vi "CalVEIN Main.vi"() -> ()   [LabVIEW 2017]
uses:
  Type Defs/Sensor Data.ctl
  Type Defs/Boxcar.ctl
panel:
  out "45% 2":string="31.00 °C"
  out "45%":string="31.10 °C"
  in  "Box cooler":bool
  out "NewVal":bool
  out "Ready To Fire Flag":bool
  out "Firing State":string[](array[string])=["System Is Not Armed", "", "", "", "", " "]
  in  "Arm Flag":bool
  in  "Sample Rate (secs)":u32=1000
  out "Burn Time\nCountdown (secs)":string="0.00"
  out "Boxcar Data":T1={"AI Sensor Data"={"Sensor Array"=[{"Description"="P2 - LOX Tank Pressure", "Last Reading"="-1.72", "Coefs"=[0.0, 5000.0], "Eng Units"="psig"}, {"Description"="P3 - Fuel Tank Pressure", "Last Reading"="-1.03", "Coefs"=[0.0, 5000.0], "Eng Units"="psig"}, {"Description"="P1 - Chamber Pressure", "Last Reading"="-1.17", "Coefs"=[0.0, 5000.0], "Eng Units"="psig"}, {"Description"="Not Used", "Last Reading"="0.00", "Coefs"=[0.0, 0.0], "Eng Units"="psig"}, {"Description"="P5- DOME Reg.", "Last Reading"="-1.58", "Coefs"=[0.0, 5000.0], "Eng Units"="psig"}, {"Description"="Not Use", "Last Reading"="0.00", "Coefs"=[0.0, 0.0], "Eng Units"="psig"}, {"Description"="P4- High Pressure Tank", "Last Reading"="-1.56", "Coefs"=[0.0, 10000.0], "Eng Units"="psig"}, {"Description"="P7 - Gnd High Pressure", "Last Reading"="-4.62", "Coefs"=[0.0, 10000.0], "Eng Units"="psig"}, {"Description"="P6 - GHE Fill Pressure", "Last Reading"="2.98", "Coefs"=[0.0, 5000.0], "Eng Units"="psig"}, {"Description"="P8 - Pneumatics Pressure", "Last Reading"="0.32", "Coefs"=[0.0, 5000.0], "Eng Units"="psig"}, {"Description"="Not Used", "Last Reading"="0.00", "Coefs"=[0.0, 0.0], "Eng Units"=""}, {"Description"="Not Used", "Last Reading"="0.00", "Coefs"=[0.0, 0.0], "Eng Units"=""}, {"Description"="Not Used", "Last Reading"="0.00", "Coefs"=[0.0, 0.0], "Eng Units"=""}, {"Description"="Not Used", "Last Reading"="0.00", "Coefs"=[0.0, 0.0], "Eng Units"=""}, {"Description"="Not Used", "Last Reading"="0.00", "Coefs"=[0.0, 0.0], "Eng Units"=""}, {"Description"="Not Used", "Last Reading"="0.00", "Coefs"=[0.0, 0.0], "Eng Units"=""}, {"Description"="QD Sep Indication", "Last Reading"="5.09", "Coefs"=[0.0, 1.0], "Eng Units"="On/Off"}, {"Description"="Lift Off Indicator", "Last Reading"="5.09", "Coefs"=[0.0, 1.0], "Eng Units"="On/Off"}, {"Description"="Main Valve Open Indicator", "Last Reading"="1.79", "Coefs"=[0.0, 1.0], "Eng Units"="On/Off"}, {"Description"="Main Valve Closed Indicator", "Last Reading"="1.76", "Coefs"=[0.0, 1.0], "Eng Units"="On/Off"}, {"Description"="Load Cell 1 - Veh Gross Weight", "Last Reading"="0.13", "Coefs"=[-122.0, 8333.3], "Eng Units"="lbf"}, {"Description"="Load Cell 2 - - Veh Gross Weight", "Last Reading"="-2.48", "Coefs"=[0.0, 8333.33], "Eng Units"="lbf"}, {"Description"="Not Used", "Last Reading"="0.00", "Coefs"=[0.0, 0.0], "Eng Units"=""}, {"Description"="Not Used", "Last Reading"="0.00", "Coefs"=[0.0, 0.0], "Eng Units"=""}, {"Description"="", "Last Reading"="0.00", "Coefs"=[], "Eng Units"=""}, {"Description"="", "Last Reading"="0.00", "Coefs"=[], "Eng Units"=""}, {"Description"="", "Last Reading"="0.00", "Coefs"=[], "Eng Units"=""}, {"Description"="", "Last Reading"="0.00", "Coefs"=[], "Eng Units"=""}, {"Description"="", "Last Reading"="0.00", "Coefs"=[], "Eng Units"=""}, {"Description"="", "Last Reading"="0.00", "Coefs"=[], "Eng Units"=""}, {"Description"="", "Last Reading"="0.00", "Coefs"=[], "Eng Units"=""}, {"Description"="", "Last Reading"="0.00", "Coefs"=[], "Eng Units"=""}]}, "TC Array"=[31.195067822, 31.09588569350001, 31.09588569350001, 30.99670356499999, 31.195067822, 31.09588569350001, 31.09588569350001, 1369.6815, 1369.6815, 1369.6815, 1369.6815, 1369.6815, 1369.6815, 1369.6815]}
  out "?":string="3.07 psig"
  out "Log Refnum":refnum<file>
  out "Log Epoch":u32
  out "Log Number":i32=123
  in  "Data Log Flag":bool
  out "File Path":path
  out "Eng Data & Units":string[](array[string])=["-1.67 psig", "-1.03 psig", "-1.17 psig", "0.00 psig", "-1.58 psig", "0.00 psig", "-1.56 psig", "-4.62 psig", "3.07 psig", "0.32 psig", "0.00 ", "0.00 ", "0.00 ", "0.00 ", "0.00 ", "0.00 ", "5.09 On/Off", "5.09 On/Off", "1.79 On/Off", "1.75 On/Off", "0.13 lbf", "-2.48 lbf", "0.00 ", "0.00 ", "0.00 ", "0.00 ", "0.00 ", "0.00 ", "0.00 ", "0.00 ", "0.00 ", "0.00 "]
  out "TC String Array":string[](array[string])=["31.20 °C", "31.10 °C", "31.10 °C", "31.00 °C", "31.20 °C", "31.10 °C", "31.10 °C", "1369.68 °C", "1369.68 °C", "1369.68 °C", "1369.68 °C", "1369.68 °C", "1369.68 °C", "1369.68 °C"]
  in  "Data Log Button":bool
  in  "Sequence Abort":bool
  out "Igniter Abort":bool
  out "Elapsed Time":u32=10554
  in  "Auto Sequence":bool
  in  "Auto Sequence Flag":bool
  out "Epoch":u32=5746771
  out "Countdown (secs)":i32
  in  "MV Open Start":dbl
  in  "Burn Time":dbl=3.0
  in  "Igniter Start":dbl=-3.0
  in  "Countdown":dbl=-10.0
  in  "Igniter Minimum\nTemp (°C)":dbl=200.0
  in  "Auto Switch":bool
  out "?":string="1369.68 °C"
  out "Thermometer 2":dbl(slide)=1369.6815 scale=0.0..1000.0
  out "Thermometer":dbl(slide)=1369.6815 scale=0.0..1000.0
  out "Igniter Temp (°C)":string="1369.68 °C"
  out "?":string="31.20 °C"
  out "30%":string="31.10 °C"
  out "QD Sep Indicator":bool=TRUE
  out "Liftoff Indicator":bool=TRUE
  out "MV Closed Ind":bool
  out "MV Open Ind":bool
  out "?":string="0.13 lbf"
  out "?":string="0.32 psig"
  out "?":string="-4.62 psig"
  out "?":string="-1.58 psig"
  out "?":string="-1.56 psig"
  out "?":string="-1.17 psig"
  out "P3":string="-1.03 psig"
  in  "High Press":bool
  in  "High Press Vent":bool
  in  "MV Open":bool
  in  "MV Closed":bool
  out "P2":string="-1.67 psig"
  in  "Remote QD Sep":bool
  in  "GHe Fill":bool
  in  "Igniter Pwr":bool
  in  "Dome Reg":bool
  in  "Dome Vent":bool
  in  "Fuel Vent":bool
  in  "LOX Vent":bool
  out "Relay States":bool[](array[boolean])
  in  "stop":bool
  in  "AI Sensor Data":T2={"Sensor Array"=[{"Description"="P2 - LOX Tank Pressure", "Last Reading"="-1.67", "Coefs"=[0.0, 5000.0], "Eng Units"="psig"}, {"Description"="P3 - Fuel Tank Pressure", "Last Reading"="-1.03", "Coefs"=[0.0, 5000.0], "Eng Units"="psig"}, {"Description"="P1 - Chamber Pressure", "Last Reading"="-1.17", "Coefs"=[0.0, 5000.0], "Eng Units"="psig"}, {"Description"="Not Used", "Last Reading"="0.00", "Coefs"=[0.0, 0.0], "Eng Units"="psig"}, {"Description"="P5- DOME Reg.", "Last Reading"="-1.58", "Coefs"=[0.0, 5000.0], "Eng Units"="psig"}, {"Description"="Not Use", "Last Reading"="0.00", "Coefs"=[0.0, 0.0], "Eng Units"="psig"}, {"Description"="P4- High Pressure Tank", "Last Reading"="-1.56", "Coefs"=[0.0, 10000.0], "Eng Units"="psig"}, {"Description"="P7 - Gnd High Pressure", "Last Reading"="-4.62", "Coefs"=[0.0, 10000.0], "Eng Units"="psig"}, {"Description"="P6 - GHE Fill Pressure", "Last Reading"="3.07", "Coefs"=[0.0, 5000.0], "Eng Units"="psig"}, {"Description"="P8 - Pneumatics Pressure", "Last Reading"="0.32", "Coefs"=[0.0, 5000.0], "Eng Units"="psig"}, {"Description"="Not Used", "Last Reading"="0.00", "Coefs"=[0.0, 0.0], "Eng Units"=""}, {"Description"="Not Used", "Last Reading"="0.00", "Coefs"=[0.0, 0.0], "Eng Units"=""}, {"Description"="Not Used", "Last Reading"="0.00", "Coefs"=[0.0, 0.0], "Eng Units"=""}, {"Description"="Not Used", "Last Reading"="0.00", "Coefs"=[0.0, 0.0], "Eng Units"=""}, {"Description"="Not Used", "Last Reading"="0.00", "Coefs"=[0.0, 0.0], "Eng Units"=""}, {"Description"="Not Used", "Last Reading"="0.00", "Coefs"=[0.0, 0.0], "Eng Units"=""}, {"Description"="QD Sep Indication", "Last Reading"="5.09", "Coefs"=[0.0, 1.0], "Eng Units"="On/Off"}, {"Description"="Lift Off Indicator", "Last Reading"="5.09", "Coefs"=[0.0, 1.0], "Eng Units"="On/Off"}, {"Description"="Main Valve Open Indicator", "Last Reading"="1.79", "Coefs"=[0.0, 1.0], "Eng Units"="On/Off"}, {"Description"="Main Valve Closed Indicator", "Last Reading"="1.75", "Coefs"=[0.0, 1.0], "Eng Units"="On/Off"}, {"Description"="Load Cell 1 - Veh Gross Weight", "Last Reading"="0.13", "Coefs"=[-122.0, 8333.3], "Eng Units"="lbf"}, {"Description"="Load Cell 2 - - Veh Gross Weight", "Last Reading"="-2.48", "Coefs"=[0.0, 8333.33], "Eng Units"="lbf"}, {"Description"="Not Used", "Last Reading"="0.00", "Coefs"=[0.0, 0.0], "Eng Units"=""}, {"Description"="Not Used", "Last Reading"="0.00", "Coefs"=[0.0, 0.0], "Eng Units"=""}, {"Description"="", "Last Reading"="0.00", "Coefs"=[], "Eng Units"=""}, {"Description"="", "Last Reading"="0.00", "Coefs"=[], "Eng Units"=""}, {"Description"="", "Last Reading"="0.00", "Coefs"=[], "Eng Units"=""}, {"Description"="", "Last Reading"="0.00", "Coefs"=[], "Eng Units"=""}, {"Description"="", "Last Reading"="0.00", "Coefs"=[], "Eng Units"=""}, {"Description"="", "Last Reading"="0.00", "Coefs"=[], "Eng Units"=""}, {"Description"="", "Last Reading"="0.00", "Coefs"=[], "Eng Units"=""}, {"Description"="", "Last Reading"="0.00", "Coefs"=[], "Eng Units"=""}]}
  # "CSULB Launch Team Control System"
  # "Questions regrads this system please direct them to Thanh Truc Le truclee126@gmail.com"
  # "Autosequence\n Parameters"
  # "30%"
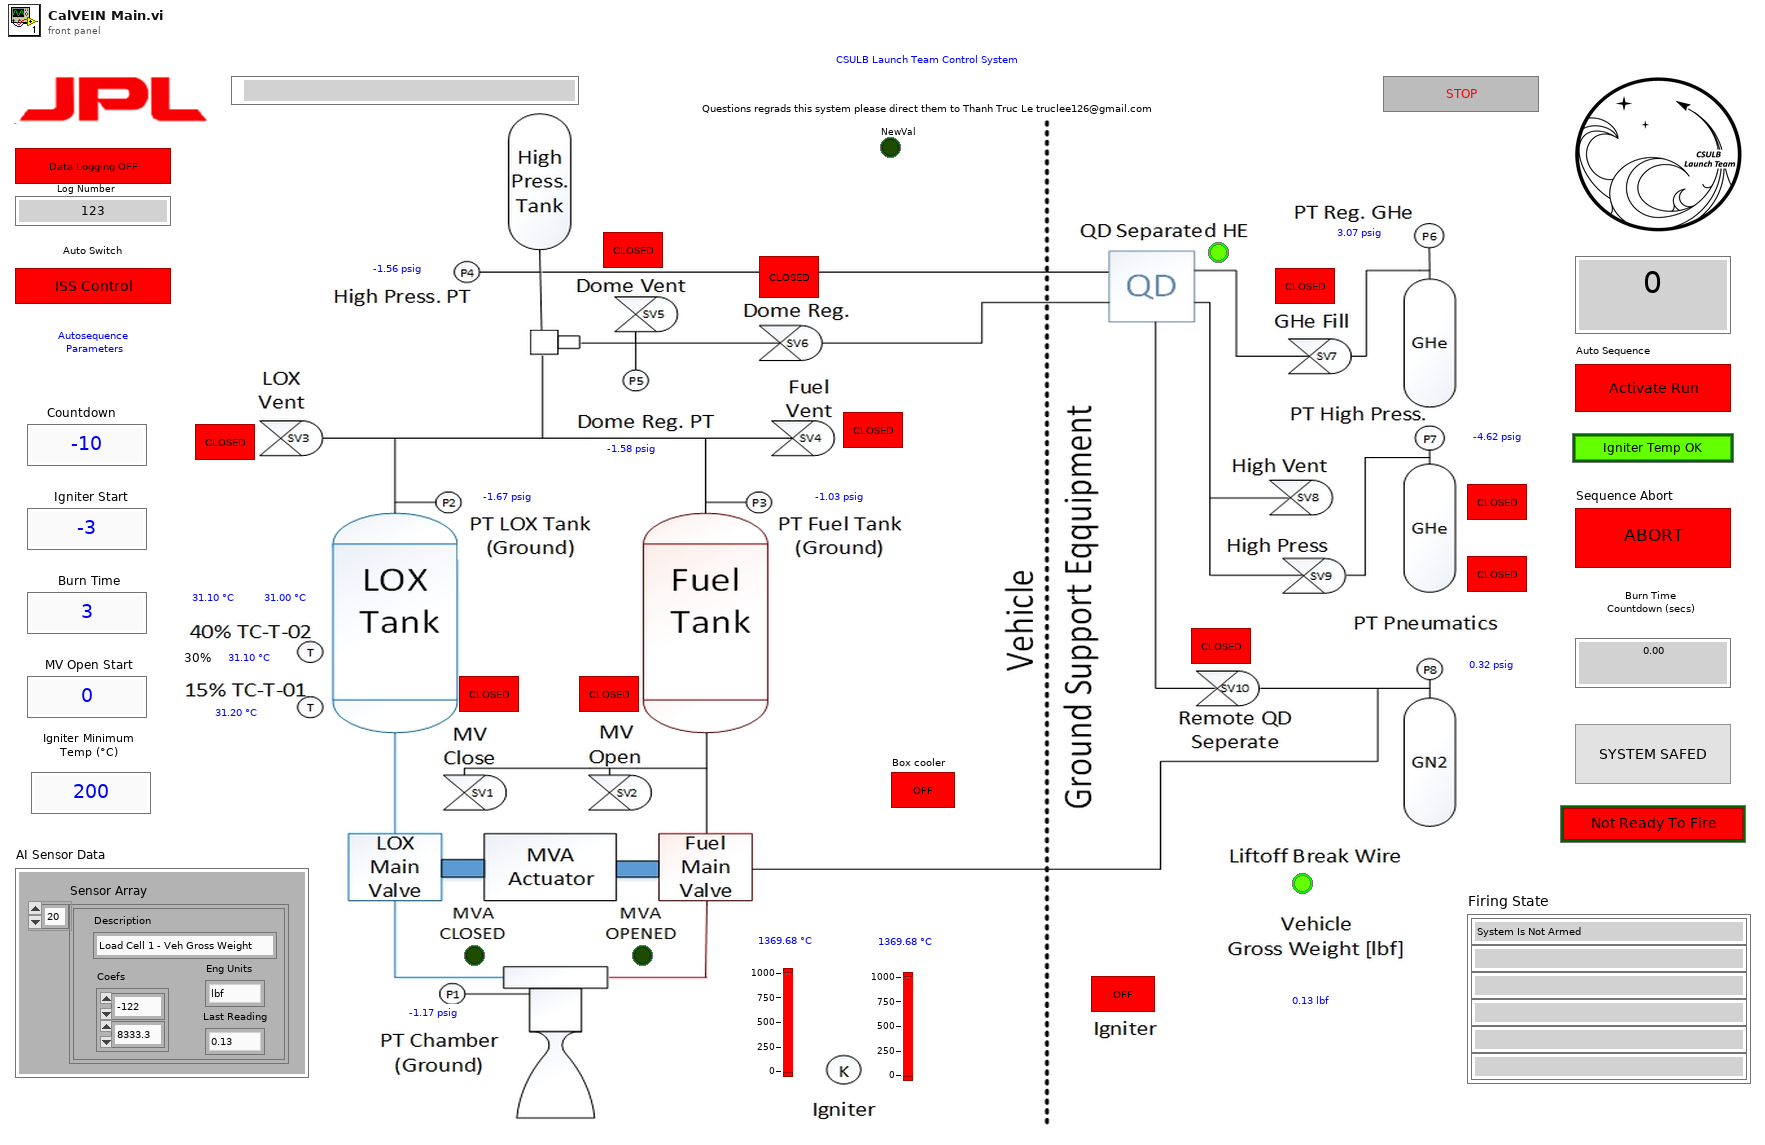
[diagram p1: front panel]
types:
  T1 = typedef "Boxcar.ctl" = cluster{"AI Sensor Data":T2, "TC Array":dbl[]}
  T2 = typedef "Sensor Data.ctl" = cluster{"Sensor Array":cluster{"Description":string, "Last Reading":string, "Coefs":dbl[], "Eng Units":string}[]}
  T3 = cluster{"Description":string, "Last Reading":string, "Coefs":dbl[], "Eng Units":string}[]
  T4 = enum16{"open", "replace", "create", "open or create", "replace or create", "replace or create with confirmation"}
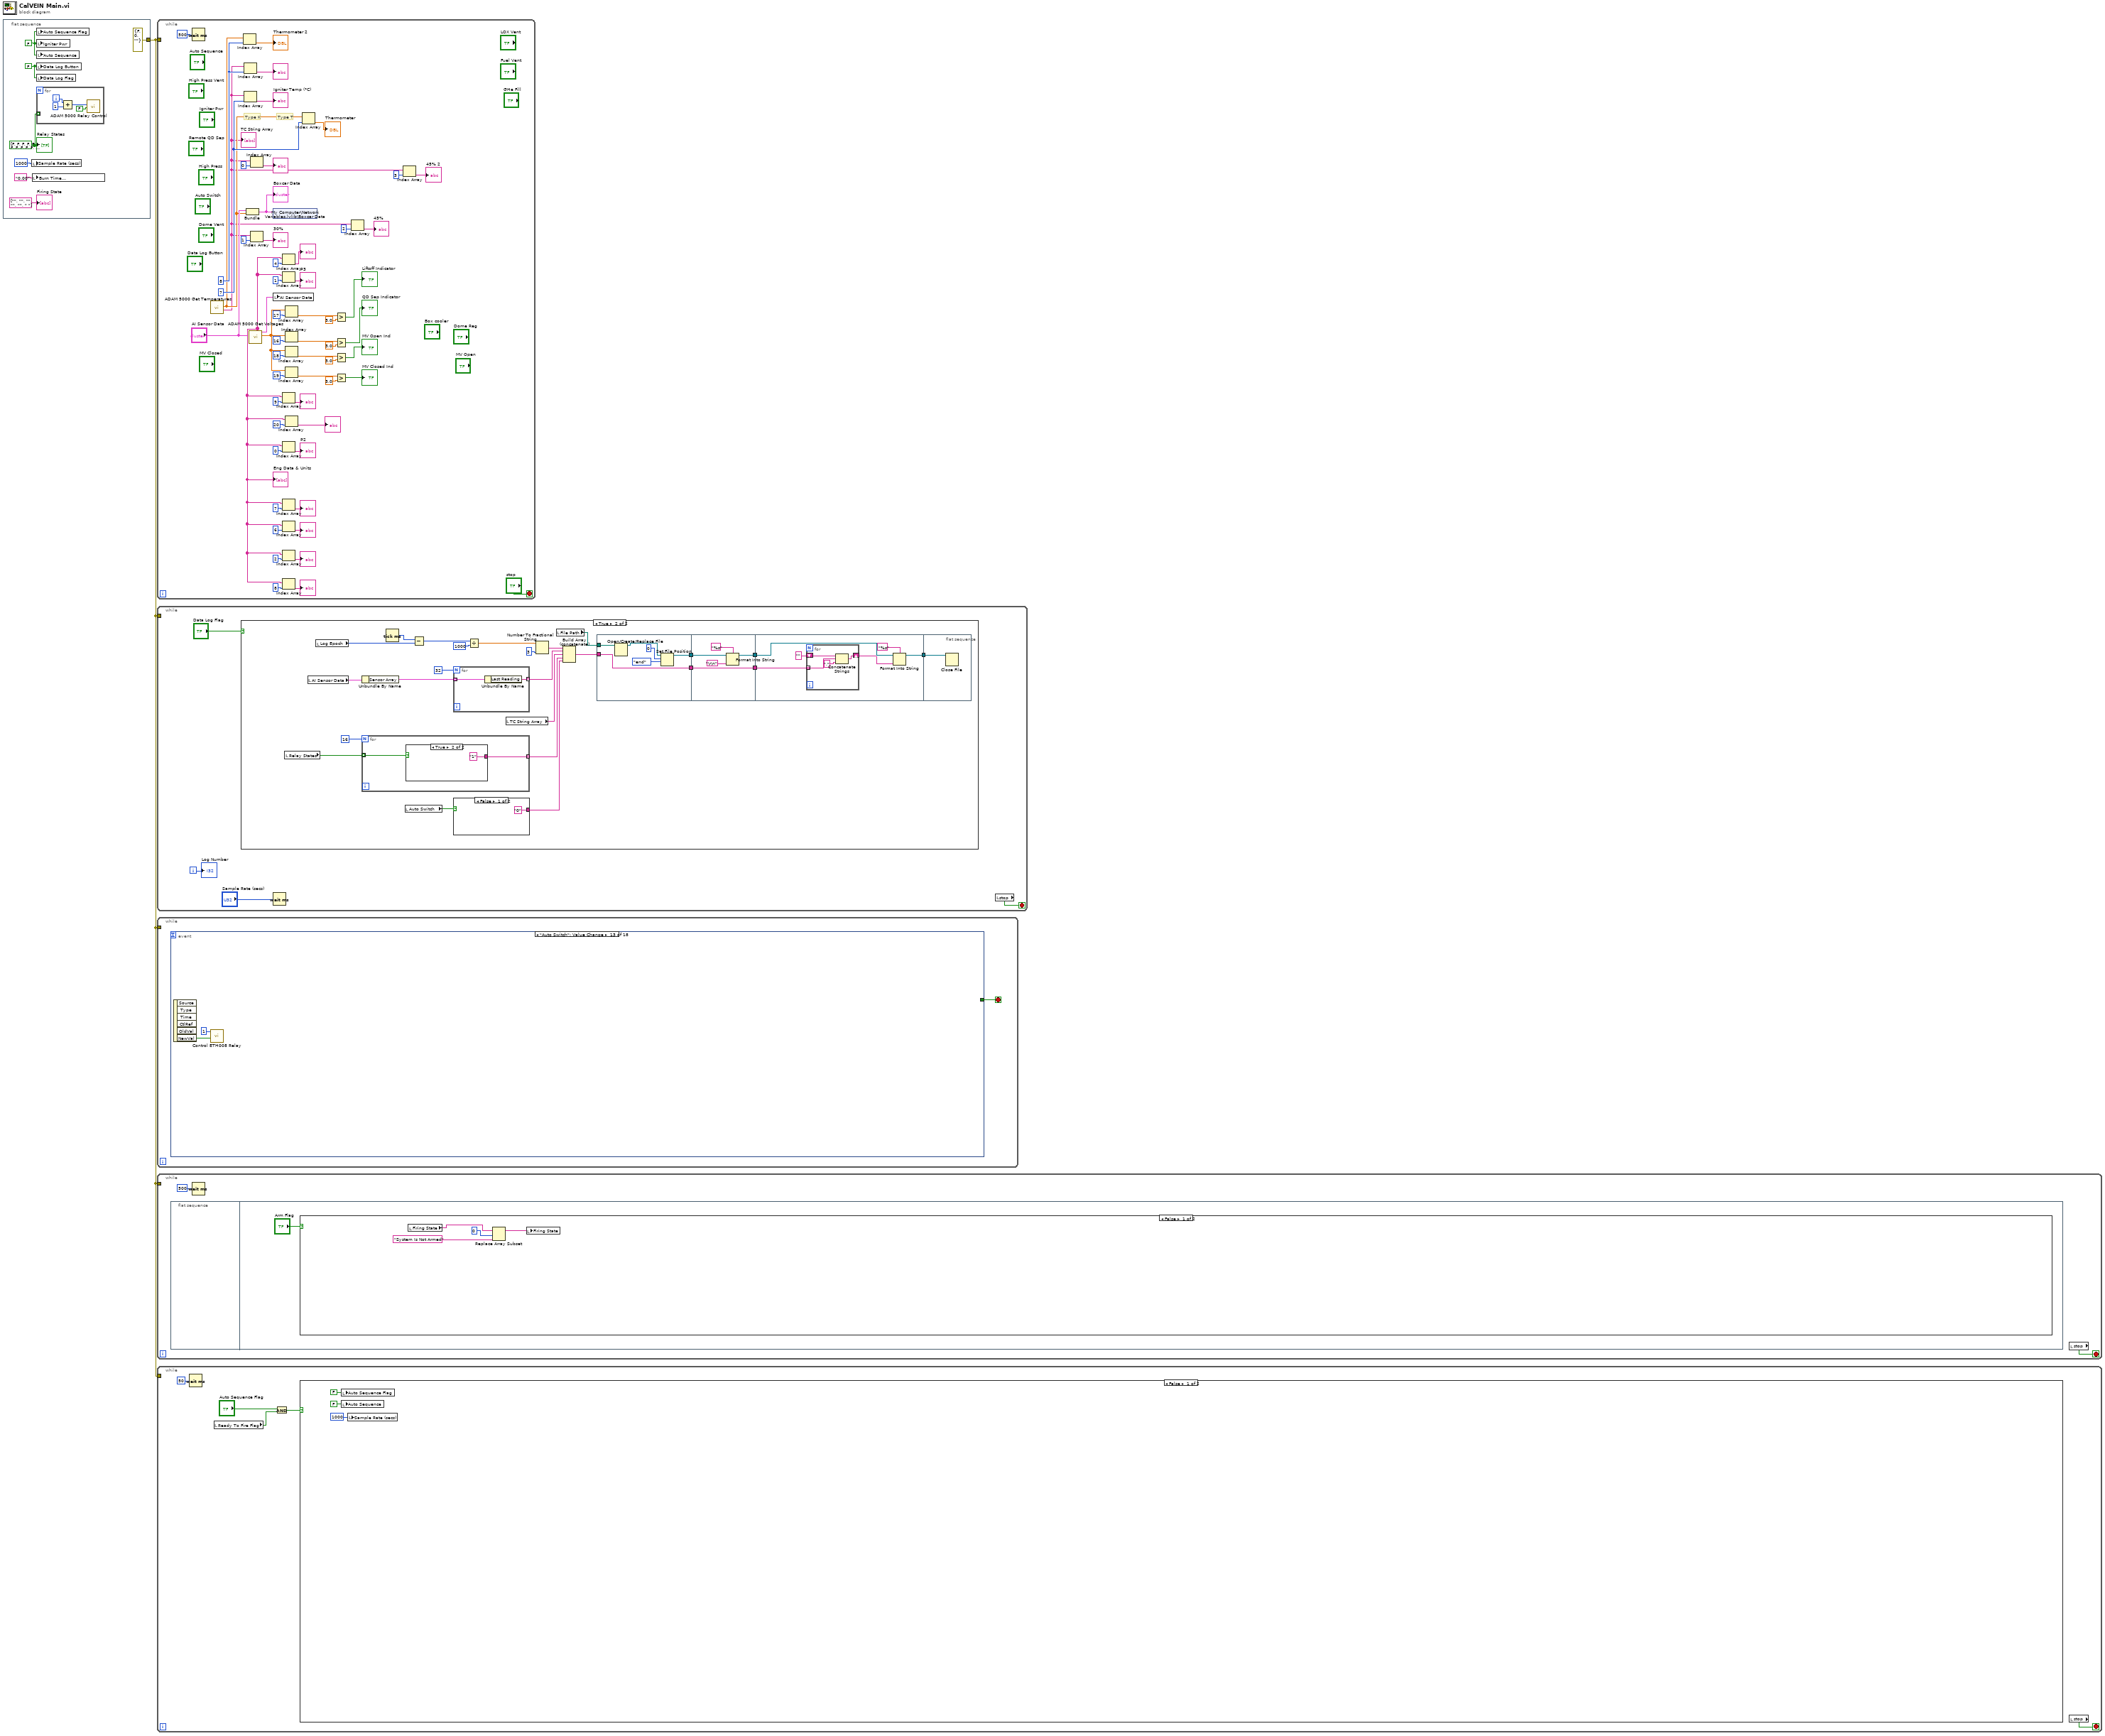
[diagram p0: block diagram]
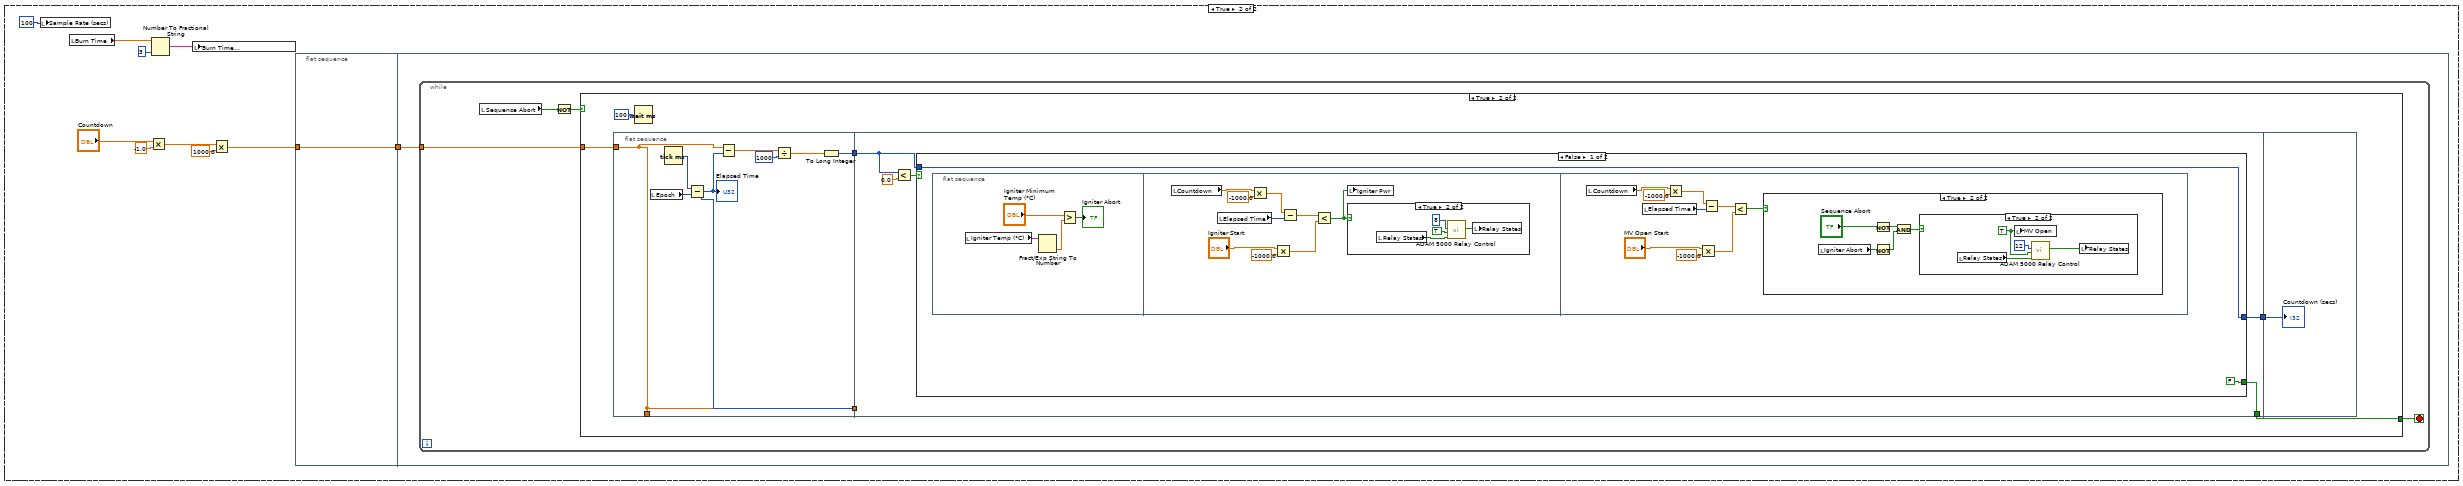
[diagram p2: hidden frame]
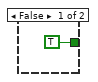
[diagram p3: hidden frame]
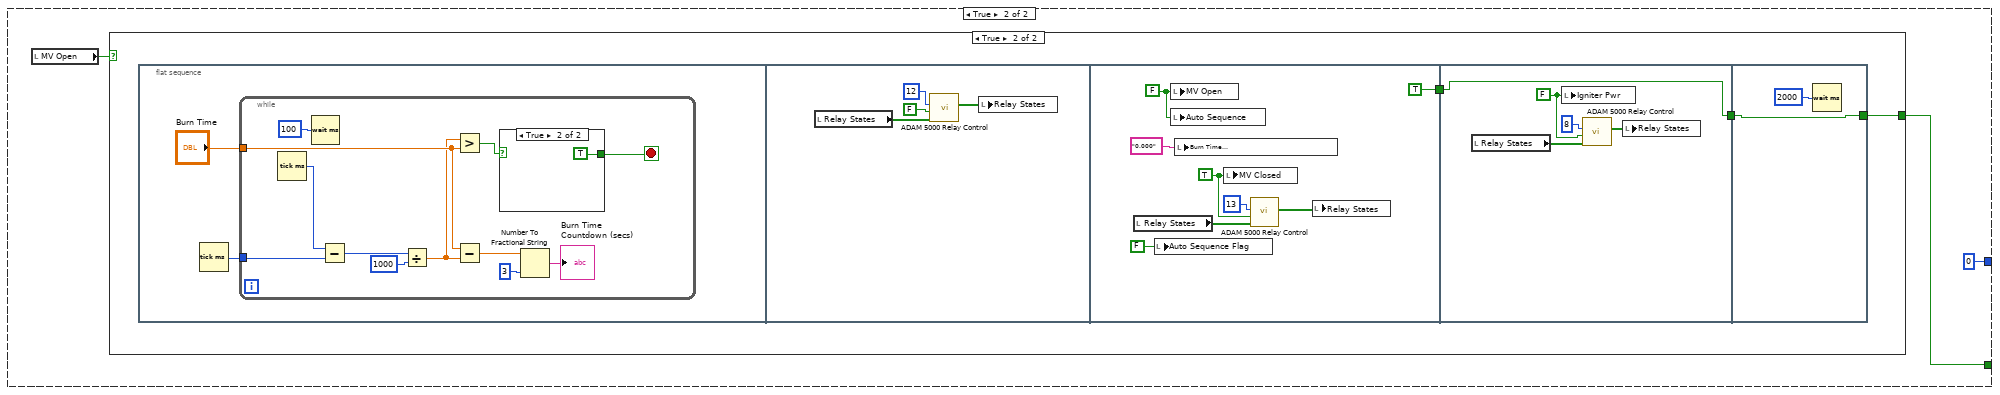
[diagram p7: hidden frame]
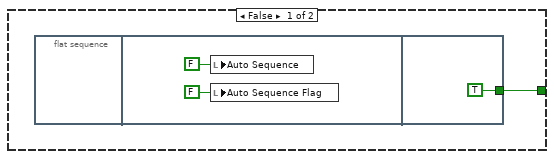
[diagram p8: hidden frame]
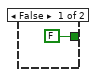
[diagram p9: hidden frame]
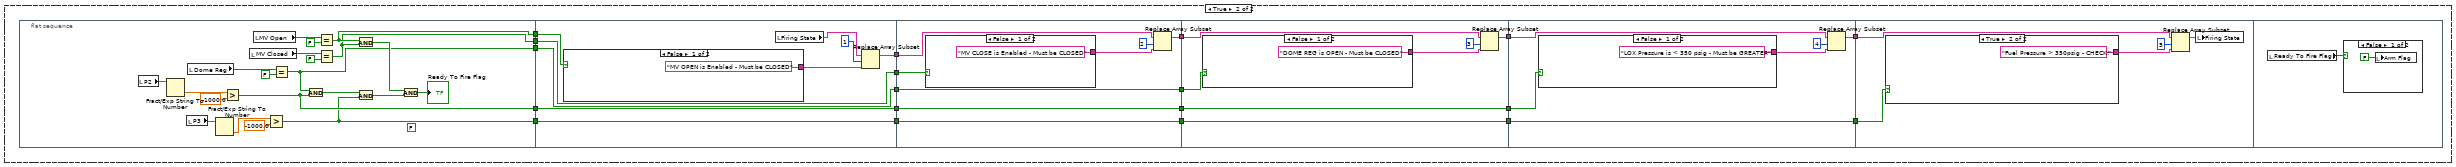
[diagram p10: hidden frame]
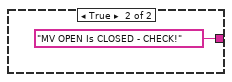
[diagram p11: hidden frame]
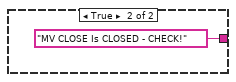
[diagram p12: hidden frame]
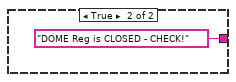
[diagram p13: hidden frame]
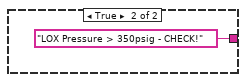
[diagram p14: hidden frame]
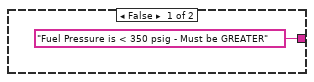
[diagram p15: hidden frame]
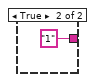
[diagram p18: hidden frame]
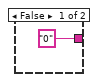
[diagram p19: hidden frame]
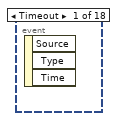
[diagram p20: hidden frame]
diagram:
  n1 = flat-sequence {
    tunnel: [errorcluster {"status"=FALSE, "code"=0, "source"=""} ("error constant")] -> w1
    frame #0 {
      w5 = FALSE ("Data Lof Flag")
      w6 = FALSE ("Auto Sequence Flag")
      w7 = bool[] [FALSE, FALSE, FALSE, FALSE, FALSE, FALSE, FALSE, FALSE, FALSE, FALSE, FALSE, FALSE, FALSE, FALSE, FALSE, FALSE]
      n2 = local write "Sample Rate (secs)"(u32 1000 ("Sample Rate (secs)")) -> ()
      n3 = local write "Burn Time\nCountdown (secs)"("0.00" ("Burn Time\nCountdown (secs)")) -> ()
      n4 = local write "Auto Sequence Flag"(w6) -> ()
      n5 = local write "Igniter Pwr"(w6) -> ()
      n6 = local write "Auto Sequence"(w6) -> ()
      n7 = local write "Data Log Button"(w5) -> ()
      n8 = local write "Data Log Flag"(w5) -> ()
      n9 = for {
        tunnel: w7 -> [_] mode=indexing
        i -> [w12]
        n10 = Add(x=w12, y=1) -> (x+y=w10:i32)
        n11 = call "ADAM 5000 Relay Control.vi"("State"=FALSE, "Relay # (1=1st relay)"=w10) -> ()  [unwired: 9 in, 1 out]
      }
      "Relay States" <- w7
      "Firing State" <- string[] ["", "", "", "", "", " "]
    }
  }
  n12 = while {
    tunnel: w1 -> [_]
    stop <- "stop" stop-if-true
    w25 = 8 ("index")
    w28 = 7 ("index")
    # "Type T"
    # "Type K"
    n13 = Wait (ms)(milliseconds to wait=u32 500) -> ()  [unwired: 1 out]
    n14 = call "ADAM 5000 Get Temperatures.vi"() -> ("TC String Array"=w13:string[], "TC Array"=w19:dbl[])  [unwired: 10 in]
    "TC String Array" <- w13
    n15 = Index Array(array=w19, index=w25) -> (element=→"Thermometer 2":dbl)
    n16 = Index Array(array=w13, index=w25) -> (element=→"?":string)
    n17 = Index Array(array=w13, index=w28) -> (element=→"Igniter Temp (°C)":string)
    n18 = Bundle("AI Sensor Data"="AI Sensor Data", "TC Array"=w19) -> (w18:cluster{"AI Sensor Data":T2, "TC Array":dbl[]})  [unwired: 1 in]
    "Boxcar Data" <- w18
    n19 = call "ADAM 5000 Get Voltages.vi"("AI Sensor Data"="AI Sensor Data") -> ("Master Raw Data Vdc"=w34:dbl[], "AI Sensor Data Out"=w67:T2, "Eng Data & Units"=w21:string[])  [unwired: 5 in, 3 out]
    "Eng Data & Units" <- w21
    n20 = Index Array(array=w13, index=0) -> (element=→"?":string)
    n21 = Index Array(array=w13, index=1) -> (element=→"30%":string)
    n22 = shared-variable "My Computer\\Network Variables.lvlib\\Boxcar Data"(w18) -> ()  [unwired: 1 in, 1 out]
    n23 = local write "AI Sensor Data"(w67) -> ()
    n24 = Index Array(array=w21, index=4) -> (element=→"?":string)
    n25 = Index Array(array=w21, index=1) -> (element=→"P3":string)
    n26 = Index Array(array=w21, index=9) -> (element=→"?":string)
    n27 = Index Array(array=w21, index=0) -> (element=→"P2":string)
    n28 = Index Array(array=w21, index=7) -> (element=→"?":string)
    n29 = Index Array(array=w21, index=6) -> (element=→"?":string)
    n30 = Index Array(array=w21, index=2) -> (element=→"?":string)
    n31 = Index Array(array=w21, index=8) -> (element=→"?":string)
    n32 = Index Array(array=w34, index=17) -> (element=w41:dbl)
    n33 = Index Array(array=w34, index=16) -> (element=w36:dbl)
    n34 = Index Array(array=w34, index=18) -> (element=w49:dbl)
    n35 = Index Array(array=w34, index=19) -> (element=w45:dbl)
    n36 = Index Array(array=w21, index=20) -> (element=→"?":string)
    n37 = Index Array(array=w19, index=w28) -> (element=→"Thermometer":dbl)
    n38 = Greater?(x=w41, y=3.0) -> (0:→"Liftoff Indicator":bool)
    n39 = Greater?(x=w36, y=3.0) -> (0:→"QD Sep Indicator":bool)
    n40 = Greater?(x=w49, y=3.0) -> (0:→"MV Open Ind":bool)
    n41 = Greater?(x=w45, y=3.0) -> (0:→"MV Closed Ind":bool)
    n42 = Index Array(array=w13, index=2) -> (element=→"45%":string)
    n43 = Index Array(array=w13, index=3) -> (element=→"45% 2":string)
  }
  n44 = while {
    tunnel: w1 -> [_]
    i -> [w71]
    stop <- w73 stop-if-true
    n45 = case shown="True" "Data Log Flag" {
      frame False {
      }
      frame True {
        n46 = local read "Relay States"() -> (w95:bool[])
        n47 = local read "AI Sensor Data"() -> (w97:T2)
        n48 = local read "Log Epoch"() -> (w88:u32)
        n49 = Unbundle By Name(w97) -> ("Sensor Array"=w96:T3)
        n50 = for {
          N: 16 -> [_]
          tunnel: w95 -> [w123] mode=indexing
          tunnel: [w122] -> w91 mode=indexing
          n51 = case shown="True" w123 {
            tunnel: ["0" "1"] -> w122
            frame False {
            }
            frame True {
            }
          }
        }
        n52 = Tick Count (ms)() -> (millisecond timer value=w89:u32)
        n53 = local read "Auto Switch"() -> (w94:bool)
        n54 = Subtract(x=w89, y=w88) -> (x-y=w87:u32)
        n55 = for {
          N: 32 -> [_]
          tunnel: w96 -> [w127] mode=indexing
          tunnel: [w126] -> w93 mode=indexing
          n56 = Unbundle By Name(w127) -> ("Last Reading"=w126:string)
        }
        n57 = case shown="False" w94 {
          tunnel: ["0" "1"] -> w90
          frame False {
          }
          frame True {
          }
        }
        n58 = Divide(x=w87, y=u32 1000) -> (x/y=w85:dbl)
        n59 = local read "TC String Array"() -> (w92:string[])
        n60 = Number To Fractional String(number=w85, precision (6)=i16 3) -> (F-format string=w83:string)  [unwired: 2 in]
        n61 = local read "File Path"() -> (w82:path)
        n62 = Build Array (concatenate)(w83, w93, w92, w91, w90) -> (w81:string[])
        n63 = flat-sequence {
          tunnel: w81 -> [w103]
          tunnel: w82 -> [w102]
          tunnel: [w103] -> w79
          tunnel: [w98] -> w76
          tunnel: [w104] -> w80
          tunnel: w79 -> [w108]
          tunnel: [w108] -> w78
          tunnel: w76 -> [w105]
          tunnel: w80 -> [w111]
          tunnel: w78 -> [w114]
          tunnel: [w109] -> w77
          tunnel: w77 -> [w119]
          frame #0 {
            n64 = Open/Create/Replace File(file path (use dialog)=w102) -> (refnum out=w101:refnum<file>)  [unwired: 5 in, 2 out]
            n65 = Set File Position(offset (in bytes) (0)=i64 0, refnum=w101, from (0:start)=enum16{"start", "end", "current"}."end") -> (refnum out=w98:refnum<file>)  [unwired: 1 in, 1 out]
          }
          frame #1 {
            n66 = Format Into String(format string="%s", initial string=w105, "\r\n") -> (resulting string=w104:refnum<file>)  [unwired: 1 in, 1 out]
          }
          frame #2 {
            n67 = for {
              shift-right: [w116] -> w110
              shift-left: "" -> [w115]
              tunnel: w114 -> [w118] mode=indexing
              n68 = Concatenate Strings(w115, w118, "," ("string")) -> (w116:string)
            }
            n69 = Format Into String(format string="%s", initial string=w111, w110) -> (resulting string=w109:refnum<file>)  [unwired: 1 in, 1 out]
          }
          frame #3 {
            n70 = Close File(refnum=w119) -> ()  [unwired: 1 in, 2 out]
          }
        }
      }
    }
    n71 = Wait (ms)(milliseconds to wait="Sample Rate (secs)") -> ()  [unwired: 1 out]
    n72 = local read "stop"() -> (w73:bool)
    "Log Number" <- w71
  }
  n73 = while {
    tunnel: w1 -> [_]
    stop <- w128 stop-if-true
    n74 = event shown="[12] \"Auto Switch\": Value Change" {
      selector: _ -> [_ _ _ _ _ _ _ _ _ _ _ _ _ _ _ _ _ _]
      dyn-events: _ -> [_ _ _ _ _ _ _ _ _ _ _ _ _ _ _ _ _ _]
      timeout: _ -> [_ _ _ _ _ _ _ _ _ _ _ _ _ _ _ _ _ _]
      tunnel: [_ _ _ _ _ _ _ _ w157 _ _ _ _ _ _ _ _ _] -> w128
      event Timeout {
        n75 = event-data() -> ()  [unwired: 1 in, 3 out]
      }
      event "LOX Vent": Value Change {
        n76 = event-data() -> ("NewVal"=w131:bool)  [unwired: 1 in, 5 out]
        n77 = local read "Relay States"() -> (w130:bool[])
        n78 = call "ADAM 5000 Relay Control.vi"("Relay States IN"=w130, "State"=w131, "Relay # (1=1st relay)"=1) -> ("Relay States OUT"=w129:bool[])  [unwired: 8 in]
        n79 = local write "Relay States"(w129) -> ()
      }
      event "Fuel Vent": Value Change {
        n80 = event-data() -> ("NewVal"=w133:bool)  [unwired: 1 in, 5 out]
        n81 = local read "Relay States"() -> (w135:bool[])
        n82 = call "ADAM 5000 Relay Control.vi"("Relay States IN"=w135, "State"=w133, "Relay # (1=1st relay)"=2) -> ("Relay States OUT"=w134:bool[])  [unwired: 8 in]
        n83 = local write "Relay States"(w134) -> ()
      }
      event "Dome Vent": Value Change {
        n84 = event-data() -> ("NewVal"=w137:bool)  [unwired: 1 in, 5 out]
        n85 = local read "Relay States"() -> (w139:bool[])
        n86 = call "ADAM 5000 Relay Control.vi"("Relay States IN"=w139, "State"=w137, "Relay # (1=1st relay)"=6) -> ("Relay States OUT"=w138:bool[])  [unwired: 8 in]
        n87 = local write "Relay States"(w138) -> ()
      }
      event "Dome Reg": Value Change {
        n88 = event-data() -> ("NewVal"=w141:bool)  [unwired: 1 in, 5 out]
        n89 = local read "Relay States"() -> (w143:bool[])
        n90 = call "ADAM 5000 Relay Control.vi"("Relay States IN"=w143, "State"=w141, "Relay # (1=1st relay)"=5) -> ("Relay States OUT"=w142:bool[])  [unwired: 8 in]
        n91 = local write "Relay States"(w142) -> ()
      }
      event "Igniter Pwr": Value Change {
        n92 = event-data() -> ("NewVal"=w145:bool)  [unwired: 1 in, 5 out]
        n93 = local read "Relay States"() -> (w147:bool[])
        n94 = call "ADAM 5000 Relay Control.vi"("Relay States IN"=w147, "State"=w145, "Relay # (1=1st relay)"=8) -> ("Relay States OUT"=w146:bool[])  [unwired: 8 in]
        n95 = local write "Relay States"(w146) -> ()
      }
      event "GHe Fill": Value Change {
        n96 = event-data() -> ("NewVal"=w149:bool)  [unwired: 1 in, 5 out]
        n97 = local read "Relay States"() -> (w151:bool[])
        n98 = call "ADAM 5000 Relay Control.vi"("Relay States IN"=w151, "State"=w149, "Relay # (1=1st relay)"=9) -> ("Relay States OUT"=w150:bool[])  [unwired: 8 in]
        n99 = local write "Relay States"(w150) -> ()
      }
      event "Remote QD Sep": Value Change {
        n100 = event-data() -> ("NewVal"=w153:bool)  [unwired: 1 in, 5 out]
        n101 = local read "Relay States"() -> (w155:bool[])
        n102 = call "ADAM 5000 Relay Control.vi"("Relay States IN"=w155, "State"=w153, "Relay # (1=1st relay)"=10) -> ("Relay States OUT"=w154:bool[])  [unwired: 8 in]
        n103 = local write "Relay States"(w154) -> ()
      }
      event "stop": Value Change {
        n104 = event-data() -> ()  [unwired: 1 in, 6 out]
        n105 = flat-sequence {
          tunnel: [TRUE] -> w157
          frame #0 {
            n106 = Wait (ms)(milliseconds to wait=u32 2000) -> ()  [unwired: 1 out]
          }
          frame #1 {
          }
        }
      }
      event "MV Closed": Value Change {
        n107 = event-data() -> ("NewVal"=w160:bool)  [unwired: 1 in, 5 out]
        n108 = local read "Relay States"() -> (w162:bool[])
        n109 = call "ADAM 5000 Relay Control.vi"("Relay States IN"=w162, "State"=w160, "Relay # (1=1st relay)"=13) -> ("Relay States OUT"=w161:bool[])  [unwired: 8 in]
        n110 = local write "Relay States"(w161) -> ()
      }
      event "High Press Vent": Value Change {
        n111 = event-data() -> ("NewVal"=w164:bool)  [unwired: 1 in, 5 out]
        n112 = local read "Relay States"() -> (w166:bool[])
        n113 = call "ADAM 5000 Relay Control.vi"("Relay States IN"=w166, "State"=w164, "Relay # (1=1st relay)"=15) -> ("Relay States OUT"=w165:bool[])  [unwired: 8 in]
        n114 = local write "Relay States"(w165) -> ()
      }
      event "High Press": Value Change {
        n115 = event-data() -> ("NewVal"=w168:bool)  [unwired: 1 in, 5 out]
        n116 = local read "Relay States"() -> (w170:bool[])
        n117 = call "ADAM 5000 Relay Control.vi"("Relay States IN"=w170, "State"=w168, "Relay # (1=1st relay)"=7) -> ("Relay States OUT"=w169:bool[])  [unwired: 8 in]
        n118 = local write "Relay States"(w169) -> ()
      }
      event "Auto Switch": Value Change {
        n119 = event-data() -> ("NewVal"=w173:bool)  [unwired: 1 in, 5 out]
        n120 = call "Control ETH008 Relay.vi"("On/Off"=w173, "Relay Number"=1) -> ()  [unwired: 10 in]
      }
      event "Auto Sequence": Value Change {
        w174 = TRUE ("Auto Sequence Flag")
        n121 = event-data() -> ()  [unwired: 1 in, 6 out]
        n122 = Tick Count (ms)() -> (millisecond timer value=→"Epoch":u32)
        n123 = local write "Auto Sequence Flag"(w174) -> ()
        n124 = local write "Auto Sequence"(w174) -> ()
      }
      event "Sequence Abort": Value Change {
        n125 = event-data() -> ()  [unwired: 1 in, 6 out]
        n126 = flat-sequence {
          frame #0 {
            w176 = FALSE ("Auto Sequence Flag")
            n127 = local write "Auto Sequence Flag"(w176) -> ()
            n128 = local write "Igniter Pwr"(w176) -> ()
            n129 = local write "Auto Sequence"(w176) -> ()
          }
          frame #1 {
            n130 = for {
              tunnel: bool[] [FALSE, FALSE, FALSE, FALSE, FALSE, FALSE, FALSE, FALSE, FALSE, FALSE, FALSE, FALSE, FALSE, FALSE, FALSE, FALSE] -> [_] mode=indexing
              i -> [w181]
              n131 = Add(x=w181, y=1) -> (x+y=w179:i32)
              n132 = call "ADAM 5000 Relay Control.vi"("State"=FALSE, "Relay # (1=1st relay)"=w179) -> ()  [unwired: 9 in, 1 out]
            }
          }
        }
      }
      event "Data Log Button": Value Change {
        n133 = event-data() -> ("NewVal"=w182:bool)  [unwired: 1 in, 5 out]
        n134 = case shown="True" w182 {
          frame False {
            n135 = local write "Data Log Flag"(FALSE ("Data Lof Flag")) -> ()
            n136 = local write "Data Log Flag"(FALSE ("Data Lof Flag")) -> ()
            n137 = local write "Data Log Flag"(FALSE ("Data Lof Flag")) -> ()
            n138 = local write "Data Log Flag"(FALSE ("Data Lof Flag")) -> ()
            n139 = local write "Data Log Flag"(FALSE ("Data Lof Flag")) -> ()
            n140 = local write "Data Log Flag"(FALSE ("Data Lof Flag")) -> ()
            n141 = local write "Data Log Flag"(FALSE ("Data Lof Flag")) -> ()
            n142 = local write "Data Log Flag"(FALSE ("Data Lof Flag")) -> ()
            n143 = local write "Data Log Flag"(FALSE ("Data Lof Flag")) -> ()
            n144 = local write "Data Log Flag"(FALSE ("Data Lof Flag")) -> ()
            n145 = local write "Data Log Flag"(FALSE ("Data Lof Flag")) -> ()
          }
          frame True {
            n146 = flat-sequence {
              frame #0 {
                n147 = Tick Count (ms)() -> (millisecond timer value=→"Log Epoch":u32)
                n148 = for {
                  N: 14 -> [_]
                  tunnel: [w226] -> w205 mode=indexing
                  i -> [w225]
                  n149 = Add(x=w225, y=1) -> (x+y=w223:i32)
                  n150 = Number To Fractional String(number=w223, precision (6)=i16 0) -> (F-format string=w227:string)  [unwired: 2 in]
                  n151 = Concatenate Strings("TC", w227) -> (w226:string)
                }
                n152 = for {
                  N: 16 -> [_]
                  tunnel: [w219] -> w204 mode=indexing
                  i -> [w218]
                  n153 = Add(x=w218, y=1) -> (x+y=w216:i32)
                  n154 = Number To Fractional String(number=w216, precision (6)=i16 0) -> (F-format string=w220:string)  [unwired: 2 in]
                  n155 = Concatenate Strings("Relay", w220) -> (w219:string)
                }
                n156 = local read "AI Sensor Data"() -> (w211:T2)
                n157 = Unbundle By Name(w211) -> ("Sensor Array"=w210:T3)
                n158 = for {
                  tunnel: w210 -> [w231] mode=indexing
                  tunnel: [w230] -> w208 mode=indexing
                  n159 = Unbundle By Name(w231) -> ("Description"=w230:string)
                }
                n160 = Build Array (concatenate)("Time (s)", w208, w205, w204, "Manual/Auto (1=Auto)") -> (w200:string[])
                n161 = for {
                  shift-right: [w213] -> w198
                  shift-left: "" -> [w212]
                  tunnel: w200 -> [w215] mode=indexing
                  n162 = Concatenate Strings(w212, w215, "," ("string")) -> (w213:string)
                }
                n163 = Open/Create/Replace File(operation (0:open)=T4."replace or create") -> (refnum out=w197:refnum<file>)  [unwired: 5 in, 2 out]
                "Log Refnum" <- w197
                n164 = Refnum to Path(1:w197) -> (0:→"File Path":path)
                n165 = Format Into String(format string="%s", initial string=w197, w198) -> (resulting string=w194:refnum<file>)  [unwired: 1 in, 1 out]
                n166 = Close File(refnum=w194) -> ()  [unwired: 1 in, 2 out]
              }
              frame #1 {
                n167 = Wait (ms)(milliseconds to wait=u32 1000) -> ()  [unwired: 1 out]
              }
              frame #2 {
                n168 = local write "Data Log Flag"(TRUE ("Data Lof Flag")) -> ()
              }
            }
          }
        }
      }
      event "MV Open": Value Change {
        n169 = event-data() -> ("NewVal"=w237:bool)  [unwired: 1 in, 5 out]
        "NewVal" <- w237
        n170 = local read "Relay States"() -> (w235:bool[])
        n171 = call "ADAM 5000 Relay Control.vi"("Relay States IN"=w235, "State"=w237, "Relay # (1=1st relay)"=12) -> ("Relay States OUT"=w236:bool[])  [unwired: 8 in]
        n172 = local write "Relay States"(w236) -> ()
      }
      event "Box cooler": Value Change {
        n173 = event-data() -> ("NewVal"=w238:bool)  [unwired: 1 in, 5 out]
        n174 = local read "Relay States"() -> (w240:bool[])
        n175 = call "ADAM 5000 Relay Control.vi"("Relay States IN"=w240, "State"=w238, "Relay # (1=1st relay)"=3) -> ("Relay States OUT"=w241:bool[])  [unwired: 8 in]
        n176 = local write "Relay States"(w241) -> ()
      }
    }
  }
  n177 = while {
    tunnel: w1 -> [_]
    stop <- w242 stop-if-true
    n178 = flat-sequence {
      frame #0 {
      }
      frame #1 {
        n179 = case shown="False" "Arm Flag" {
          frame False {
            n180 = local read "Firing State"() -> (w248:string[])
            n181 = Replace Array Subset(array=w248, new element="System Is Not Armed" ("new element/subarray"), index=0) -> (w245:string[])
            n182 = local write "Firing State"(w245) -> ()
          }
          frame True {
            n183 = flat-sequence {
              tunnel: [w272] -> w267
              tunnel: [w271] -> w265
              tunnel: [w270] -> w261
              tunnel: [w269] -> w255
              tunnel: [w268] -> w250
              tunnel: w267 -> [w297]
              tunnel: [w293] -> w266
              tunnel: w265 -> [w293]
              tunnel: [w292] -> w264
              tunnel: [w291] -> w262
              tunnel: w261 -> [w291]
              tunnel: [w290] -> w256
              tunnel: w255 -> [w290]
              tunnel: [w289] -> w251
              tunnel: w250 -> [w289]
              tunnel: w266 -> [w305]
              tunnel: w264 -> [w304]
              tunnel: [w303] -> w263
              tunnel: w262 -> [w303]
              tunnel: [w302] -> w260
              tunnel: [w301] -> w257
              tunnel: w256 -> [w301]
              tunnel: [w300] -> w252
              tunnel: w251 -> [w300]
              tunnel: w263 -> [w314]
              tunnel: w260 -> [w313]
              tunnel: [w312] -> w259
              tunnel: [w311] -> w258
              tunnel: w257 -> [w311]
              tunnel: [w310] -> w253
              tunnel: w252 -> [w310]
              tunnel: w259 -> [w322]
              tunnel: w258 -> [w321]
              tunnel: [w320] -> w254
              tunnel: w253 -> [w320]
              tunnel: [w319] -> w249
              tunnel: w254 -> [w329]
              tunnel: w249 -> [w328]
              frame #0 {
                (unwired) FALSE ("x .and. y?")
                n184 = local read "P2"() -> (w282:string)
                n185 = Fract/Exp String To Number(string=w282) -> (number=w281:dbl)  [unwired: 3 in, 1 out]
                n186 = local read "P3"() -> (w277:string)
                n187 = local read "Dome Reg"() -> (w284:bool)
                n188 = Fract/Exp String To Number(string=w277) -> (number=w278:dbl)  [unwired: 3 in, 1 out]
                n189 = Greater?(x=w281, y=-1000.0) -> (0:w269:bool)
                n190 = local read "MV Closed"() -> (w285:bool)
                n191 = local read "MV Open"() -> (w288:bool)
                n192 = Greater?(x=w278, y=-1000.0) -> (0:w268:bool)
                n193 = Equal?(x=w284, y=FALSE) -> (x = y?=w270:bool)
                n194 = And(x=w270, y=w269) -> (x .and. y?=w276:bool)
                n195 = Equal?(x=w288, y=FALSE) -> (x = y?=w272:bool)
                n196 = Equal?(x=w285, y=FALSE) -> (x = y?=w271:bool)
                n197 = And(x=w272, y=w271) -> (x .and. y?=w275:bool)
                n198 = And(x=w276, y=w268) -> (x .and. y?=w274:bool)
                n199 = And(x=w275, y=w274) -> (x .and. y?=→"Ready To Fire Flag":bool)
              }
              frame #1 {
                n200 = case shown="False" w297 {
                  tunnel: ["MV OPEN is Enabled - Must be CLOSED" "MV OPEN Is CLOSED - CHECK!"] -> w294
                  frame False {
                  }
                  frame True {
                  }
                }
                n201 = local read "Firing State"() -> (w296:string[])
                n202 = Replace Array Subset(array=w296, new element=w294, index=1) -> (w292:string[])
              }
              frame #2 {
                n203 = case shown="False" w305 {
                  tunnel: ["MV CLOSE is Enabled - Must be CLOSED" "MV CLOSE Is CLOSED - CHECK!"] -> w307
                  frame False {
                  }
                  frame True {
                  }
                }
                n204 = Replace Array Subset(array=w304, new element=w307, index=2) -> (w302:string[])
              }
              frame #3 {
                n205 = case shown="False" w314 {
                  tunnel: ["DOME REG is OPEN - Must be CLOSED" "DOME Reg is CLOSED - CHECK!"] -> w315
                  frame False {
                  }
                  frame True {
                  }
                }
                n206 = Replace Array Subset(array=w313, new element=w315, index=3) -> (w312:string[])
              }
              frame #4 {
                n207 = case shown="False" w321 {
                  tunnel: ["LOX Pressure is < 350 psig - Must be GREATER" "LOX Pressure > 350psig - CHECK!"] -> w324
                  frame False {
                  }
                  frame True {
                  }
                }
                n208 = Replace Array Subset(array=w322, new element=w324, index=4) -> (w319:string[])
              }
              frame #5 {
                n209 = case shown="True" w329 {
                  tunnel: ["Fuel Pressure is < 350 psig - Must be GREATER" "Fuel Pressure > 350psig - CHECK!"] -> w330
                  frame False {
                  }
                  frame True {
                  }
                }
                n210 = Replace Array Subset(array=w328, new element=w330, index=5) -> (w327:string[])
                n211 = local write "Firing State"(w327) -> ()
              }
              frame #6 {
                n212 = local read "Ready To Fire Flag"() -> (w334:bool)
                n213 = case shown="False" w334 {
                  frame False {
                    n214 = local write "Arm Flag"(FALSE ("Arm Flag")) -> ()
                  }
                  frame True {
                  }
                }
              }
            }
          }
        }
      }
    }
    n215 = Wait (ms)(milliseconds to wait=u32 500) -> ()  [unwired: 1 out]
    n216 = local read "stop"() -> (w242:bool)
  }
  n217 = while {
    tunnel: w1 -> [_]
    stop <- w340 stop-if-true
    n218 = Wait (ms)(milliseconds to wait=u32 50) -> ()  [unwired: 1 out]
    n219 = local read "Ready To Fire Flag"() -> (w337:bool)
    n220 = And(x="Auto Sequence Flag", y=w337) -> (x .and. y?=w336:bool)
    n221 = case shown="False" w336 {
      frame False {
        n222 = local write "Auto Sequence Flag"(FALSE ("Auto Sequence Flag")) -> ()
        n223 = local write "Auto Sequence"(FALSE ("Auto Sequence Flag")) -> ()
        n224 = local write "Sample Rate (secs)"(u32 1000 ("Sample Rate (secs)")) -> ()
      }
      frame True {
        n225 = local write "Sample Rate (secs)"(u32 100 ("Sample Rate (secs)")) -> ()
        n226 = local read "Burn Time"() -> (w347:dbl)
        n227 = Multiply(x="Countdown", y=-1.0) -> (x*y=w348:dbl)
        n228 = Number To Fractional String(number=w347, precision (6)=i16 3) -> (F-format string=w345:string)  [unwired: 2 in]
        n229 = local write "Burn Time\nCountdown (secs)"(w345) -> ()
        n230 = Multiply(x=w348, y=1000.0) -> (x*y=w352:dbl)
        n231 = flat-sequence {
          tunnel: w352 -> [w354]
          tunnel: [w354] -> w351
          tunnel: w351 -> [w355]
          frame #0 {
          }
          frame #1 {
            n232 = while {
              tunnel: w355 -> [w359]
              stop <- w358 stop-if-true
              n233 = local read "Sequence Abort"() -> (w357:bool)
              n234 = Not(x=w357) -> (.not. x?=w356:bool)
              n235 = case shown="True" w356 {
                tunnel: w359 -> [_ w363]
                tunnel: [TRUE w361] -> w358
                frame False {
                }
                frame True {
                  n236 = flat-sequence {
                    tunnel: [w370] -> _
                    tunnel: w363 -> [w370]
                    tunnel: [w371] -> w367
                    tunnel: [w370] -> w366
                    tunnel: [w368] -> w365
                    tunnel: w367 -> [_]
                    tunnel: w366 -> [_]
                    tunnel: w365 -> [w377]
                    tunnel: [w379] -> w361
                    tunnel: [w376] -> w364
                    tunnel: w364 -> [w463]
                    frame #0 {
                      n237 = local read "Epoch"() -> (w369:u32)
                      n238 = Tick Count (ms)() -> (millisecond timer value=w375:u32)
                      n239 = Subtract(x=w375, y=w369) -> (x-y=w371:u32)
                      "Elapsed Time" <- w371
                      n240 = Subtract(x=w370, y=w371) -> (x-y=w372:dbl)
                      n241 = Divide(x=w372, y=u32 1000) -> (x/y=w373:dbl)
                      n242 = To Long Integer(number=w373) -> (32bit integer=w368:i32)
                    }
                    frame #1 {
                      n243 = Less?(x=w377, y=0.0) -> (x < y?=w378:bool)
                      n244 = case shown="False" w378 {
                        tunnel: [FALSE w420] -> w379
                        tunnel: w377 -> [w381 _]
                        tunnel: [w381 0] -> w376
                        frame False {
                          n245 = flat-sequence {
                            frame #0 {
                              n246 = local read "Igniter Temp (°C)"() -> (w386:string)
                              n247 = Fract/Exp String To Number(string=w386) -> (number=w385:dbl)  [unwired: 3 in, 1 out]
                              n248 = Greater?(x="Igniter Minimum\nTemp (°C)", y=w385) -> (0:→"Igniter Abort":bool)
                            }
                            frame #1 {
                              n249 = local read "Countdown"() -> (w395:dbl)
                              n250 = local read "Elapsed Time"() -> (w392:u32)
                              n251 = Multiply(x=w395, y=-1000.0) -> (x*y=w393:dbl)
                              n252 = Multiply(x="Igniter Start", y=-1000.0) -> (x*y=w388:dbl)
                              n253 = Subtract(x=w393, y=w392) -> (x-y=w389:dbl)
                              n254 = Less?(x=w389, y=w388) -> (x < y?=w387:bool)
                              n255 = local write "Igniter Pwr"(w387) -> ()
                              n256 = case shown="True" w387 {
                                frame False {
                                }
                                frame True {
                                n257 = local read "Relay States"() -> (w397:bool[])
                                n258 = call "ADAM 5000 Relay Control.vi"("Relay States IN"=w397, "State"=TRUE, "Relay # (1=1st relay)"=8) -> ("Relay States OUT"=w396:bool[])  [unwired: 8 in]
                                n259 = local write "Relay States"(w396) -> ()
                                }
                              }
                            }
                            frame #2 {
                              n260 = local read "Countdown"() -> (w402:dbl)
                              n261 = local read "Elapsed Time"() -> (w405:u32)
                              n262 = Multiply(x=w402, y=-1000.0) -> (x*y=w404:dbl)
                              n263 = Multiply(x="MV Open Start", y=-1000.0) -> (x*y=w408:dbl)
                              n264 = Subtract(x=w404, y=w405) -> (x-y=w407:dbl)
                              n265 = Less?(x=w407, y=w408) -> (x < y?=w400:bool)
                              n266 = case shown="True" w400 {
                                frame False {
                                }
                                frame True {
                                n267 = local read "Igniter Abort"() -> (w412:bool)
                                n268 = Not(x="Sequence Abort") -> (.not. x?=w411:bool)
                                n269 = Not(x=w412) -> (.not. x?=w410:bool)
                                n270 = And(x=w411, y=w410) -> (x .and. y?=w409:bool)
                                n271 = case shown="True" w409 {
                                frame False {
                                }
                                frame True {
                                w414 = TRUE ("State")
                                n272 = local read "Relay States"() -> (w416:bool[])
                                n273 = local write "MV Open"(w414) -> ()
                                n274 = call "ADAM 5000 Relay Control.vi"("Relay States IN"=w416, "State"=w414, "Relay # (1=1st relay)"=12) -> ("Relay States OUT"=w415:bool[])  [unwired: 8 in]
                                n275 = local write "Relay States"(w415) -> ()
                                }
                                }
                                }
                              }
                            }
                          }
                        }
                        frame True {
                          n276 = local read "MV Open"() -> (w418:bool)
                          n277 = case shown="True" w418 {
                            tunnel: [w421 w427] -> w420
                            frame False {
                              n278 = flat-sequence {
                                tunnel: [TRUE] -> w421
                                frame #0 {
                                }
                                frame #1 {
                                n279 = local write "Auto Sequence"(FALSE ("Auto Sequence Flag")) -> ()
                                n280 = local write "Auto Sequence Flag"(FALSE ("Auto Sequence Flag")) -> ()
                                }
                                frame #2 {
                                }
                              }
                            }
                            frame True {
                              n281 = flat-sequence {
                                tunnel: [TRUE] -> w426
                                tunnel: w426 -> [w460]
                                tunnel: [w460] -> w425
                                tunnel: [w462] -> w427
                                tunnel: w425 -> [w462]
                                frame #0 {
                                n282 = Tick Count (ms)() -> (millisecond timer value=w428:u32)
                                n283 = while {
                                tunnel: "Burn Time" -> [w434]
                                tunnel: w428 -> [w439]
                                stop <- w435 stop-if-true
                                n284 = Tick Count (ms)() -> (millisecond timer value=w440:u32)
                                n285 = Wait (ms)(milliseconds to wait=u32 100) -> ()  [unwired: 1 out]
                                n286 = Subtract(x=w440, y=w439) -> (x-y=w438:u32)
                                n287 = Divide(x=w438, y=u32 1000) -> (x/y=w433:dbl)
                                n288 = Greater?(x=w433, y=w434) -> (0:w436:bool)
                                n289 = Subtract(x=w434, y=w433) -> (x-y=w432:dbl)
                                n290 = case shown="True" w436 {
                                tunnel: [FALSE TRUE] -> w435
                                frame False {
                                }
                                frame True {
                                }
                                }
                                n291 = Number To Fractional String(number=w432, precision (6)=i16 3) -> (F-format string=→"Burn Time\nCountdown (secs)":string)  [unwired: 2 in]
                                }
                                }
                                frame #1 {
                                n292 = local read "Relay States"() -> (w446:bool[])
                                n293 = call "ADAM 5000 Relay Control.vi"("Relay States IN"=w446, "State"=FALSE, "Relay # (1=1st relay)"=12) -> ("Relay States OUT"=w447:bool[])  [unwired: 8 in]
                                n294 = local write "Relay States"(w447) -> ()
                                }
                                frame #2 {
                                w450 = FALSE ("Auto Sequence Flag")
                                w449 = TRUE ("State")
                                n295 = local read "Relay States"() -> (w453:bool[])
                                n296 = local write "Auto Sequence Flag"(FALSE ("Auto Sequence Flag")) -> ()
                                n297 = local write "MV Open"(w450) -> ()
                                n298 = local write "Auto Sequence"(w450) -> ()
                                n299 = local write "Burn Time\nCountdown (secs)"("0.000" ("Burn Time\nCountdown (secs)")) -> ()
                                n300 = local write "MV Closed"(w449) -> ()
                                n301 = call "ADAM 5000 Relay Control.vi"("Relay States IN"=w453, "State"=w449, "Relay # (1=1st relay)"=13) -> ("Relay States OUT"=w454:bool[])  [unwired: 8 in]
                                n302 = local write "Relay States"(w454) -> ()
                                }
                                frame #3 {
                                w456 = FALSE ("State")
                                n303 = local read "Relay States"() -> (w458:bool[])
                                n304 = local write "Igniter Pwr"(w456) -> ()
                                n305 = call "ADAM 5000 Relay Control.vi"("Relay States IN"=w458, "State"=w456, "Relay # (1=1st relay)"=8) -> ("Relay States OUT"=w457:bool[])  [unwired: 8 in]
                                n306 = local write "Relay States"(w457) -> ()
                                }
                                frame #4 {
                                n307 = Wait (ms)(milliseconds to wait=u32 2000) -> ()  [unwired: 1 out]
                                }
                              }
                            }
                          }
                        }
                      }
                    }
                    frame #2 {
                      "Countdown (secs)" <- w463
                    }
                  }
                  n308 = Wait (ms)(milliseconds to wait=u32 100) -> ()  [unwired: 1 out]
                }
              }
            }
          }
        }
      }
    }
    n309 = local read "stop"() -> (w340:bool)
  }
